vi "Parse Frame Config Data(subVI).vi"(8 "error in (no error)":errorcluster, 10 "all rows":string[][](array[string]), 11 "Config Parser BML in":refnum<class "Config Parser BML.lvclass">) -> (0 "error out":errorcluster, 1 "Pattern Name out":string, 2 "Config Data":string[](array[string]), 3 "Config Parser BML out":refnum<class "Config Parser BML.lvclass">)   [LabVIEW 2018, in "Config Parser BML.lvlib" / "Config Parser BML.lvclass"]
uses:
  Config Parser BML.lvclass
  Ctls/FRM Data - BML.ctl
  Ctls/OM - BML.ctl
  Ctls/Burst Length.ctl
  Ctls/RW Options.ctl
  Interfaces/File Parser Interface.lvlibp/Interfaces/File Parser Interface/File Parser Interface.lvclass
  C:/P4 Workspace/PC Client/Solutions/5g_eap/trunk/1.0/HiSi5GmmWave/Pattern_Gen_Tool/Interfaces/File Parser Interface.lvlibp/Interfaces/File Parser Interface/File Parser Interface.lvclass
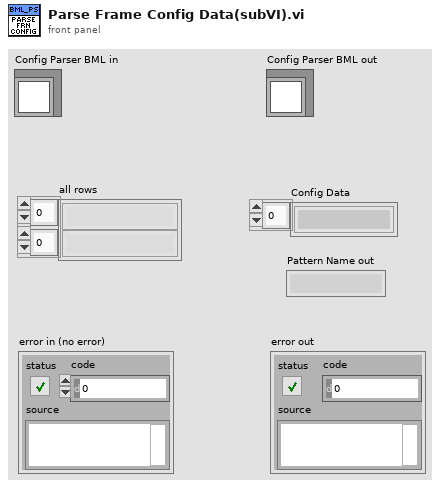
[diagram p1: front panel]
types:
  T1 = typedef "FRM Data - BML.ctl" = cluster{"Pattern_Name":string, "Data":u8[], "Start_Addr":u16, "ChipID":u8, "num of wait ms":i8, "Opcode":string[], "BML OM":T2, "BurstLength":T3, "FSN":u8, "R/W?":T4}
  T2 = typedef "OM - BML.ctl" = enum16{"Normal", "ImmeEffect", "InitSlaveID", "LoadData"}
  T3 = typedef "Burst Length.ctl" = enum8{"0", "2", "3", "4", "5", "8", "16", "32"}
  T4 = typedef "RW Options.ctl" = enum16{"Read", "Write", "R/W"}
  T5 = typedef "File Parser Interface.lvlibp/RW Options.ctl" = enum16{"Read", "Write", "R/W"}
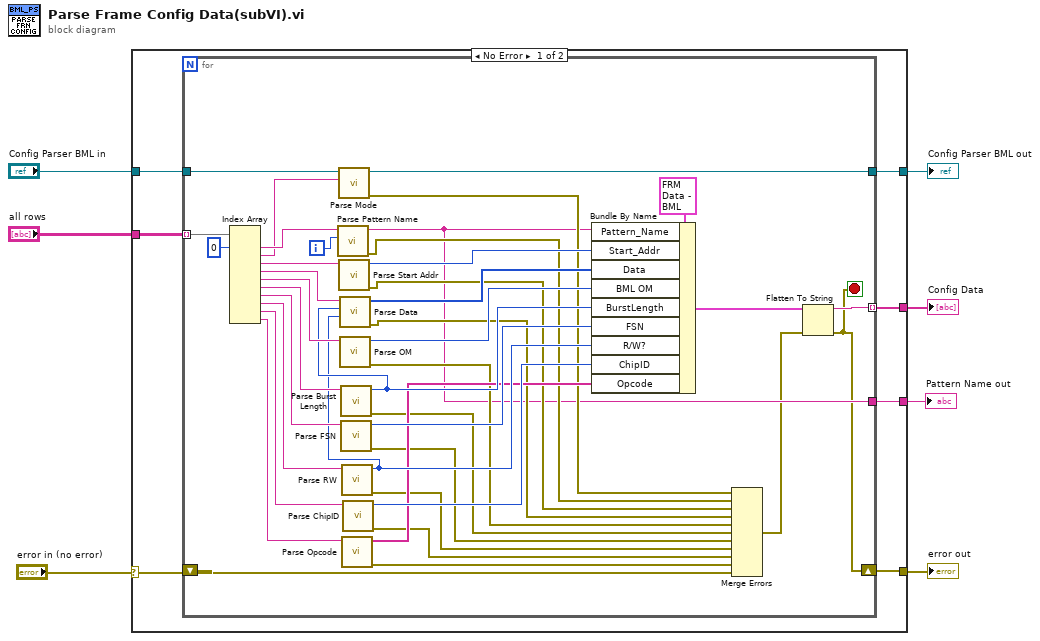
[diagram p0: block diagram]
diagram:
  n1 = case shown="No Error" "error in (no error)" {
    selector: "error in (no error)" -> [w13 w56]
    tunnel: "all rows" -> [w14 _]
    tunnel: [w12 w56] -> w5
    tunnel: [w10 w55] -> w3
    tunnel: "Config Parser BML in" -> [w11 w55]
    tunnel: [w9 _] -> w2
    tunnel: [w8 _] -> w1
    frame No Error {
      n2 = for {
        tunnel: w14 -> [w54] mode=indexing
        shift-right: [w16] -> w12
        shift-left: w13 -> [w22]
        tunnel: [w33] -> w10
        tunnel: w11 -> [w21]
        tunnel: [w19] -> w9 mode=indexing
        tunnel: [w18] -> w8
        i -> [w52]
        stop <- w16 stop-if-true
        n3 = Index Array(array=w54, index #1=0 ("index")) -> (element #1=w51:string, element #2=w34:string, element #3=w50:string, element #4=w48:string, element #5=w46:string, element #6=w44:string, element #7=w43:string, element #8=w40:string, element #9=w37:string, element #10=w35:string)  [unwired: 9 in]
        n4 = call "Parse Pattern Name.vi"("Index"=w52, "Pattern Name"=w51) -> ("error out"=w31:errorcluster, "Pattern Name out"=w18:string)  [unwired: 8 in]
        n5 = call "Parse Mode.vi"("Protocol Mode in"=w34, "File Parser Interface in"=w21) -> ("error out"=w32:errorcluster, "File Parser Interface Out"=w33:refnum<class "Config Parser BML.lvclass">)  [unwired: 8 in]
        n6 = call "Parse Start Addr.vi"("Addr in"=w50) -> ("error out"=w30:errorcluster, "Addr out"=w49:u16)  [unwired: 9 in]
        n7 = call "Parse OM.vi"("OM in"=w46) -> ("error out"=w28:errorcluster, "BML OM"=w45:T2)  [unwired: 9 in]
        n8 = call "Parse Burst Length.vi"("Burst Length in"=w44) -> ("error out"=w27:errorcluster, "BurstLength"=w42:T3)  [unwired: 9 in]
        n9 = call "Parse FSN.vi"("FSN in"=w43) -> ("error out"=w26:errorcluster, "FSN out"=w41:u8)  [unwired: 9 in]
        n10 = call "Parse RW.vi"("R/W mode in"=w40) -> ("error out"=w25:errorcluster, "R/W?"=w39:T5)  [unwired: 9 in]
        n11 = call "Parse Data.vi"("R/W?"=w39, "BurstLength"=w42, "Data in"=w48) -> ("error out"=w29:errorcluster, "Data Array out"=w47:u8[])  [unwired: 7 in]
        n12 = call "Parse Opcode.vi"("Opcode"=w35) -> ("Error out"=w23:errorcluster, "Opcode Array"=w36:string[])  [unwired: 9 in]
        n13 = call "Parse ChipID.vi"("String"=w37) -> ("error out"=w24:errorcluster, "ChipID"=w38:u8)  [unwired: 9 in]
        n14 = Bundle By Name(cluster=T1 {"Pattern_Name"="", "Data"=[], "Start_Addr"=0, "ChipID"=1, "num of wait ms"=0, "Opcode"=[], "BML OM"=enum."Normal", "BurstLength"=enum."0", "FSN"=0, "R/W?"=enum."Read"} ("Frame Data"), "Pattern_Name"=w18, "Start_Addr"=w49, "Data"=w47, "BML OM"=w45, "BurstLength"=w42, "FSN"=w41, "R/W?"=w39, "ChipID"=w38, "Opcode"=w36) -> (w20:T1)
        n15 = Merge Errors(w32, w31, w30, w29, w28, w27, w26, w25, w24, w23, w22) -> (w17:errorcluster)
        n16 = Flatten To String(anything=w20, error in (no error)=w17) -> (data string=w19:string, error out=w16:errorcluster)  [unwired: 2 in, 1 out]
      }
    }
    frame Error {
    }
  }
  "error out" <- w5
  "Config Parser BML out" <- w3
  "Config Data" <- w2
  "Pattern Name out" <- w1
